vi "Get Main Log Path and Name from Config.vi"(8 "error in":errorcluster, 11 "Main Config File Refnum":T1) -> (0 "error out":errorcluster, 1 "LogBaseName":string, 2 "LogBasePath":path)   [LabVIEW 2018]
uses:
  <vilib>/Utility/config.llb/Config Data RefNum.ctl
  <vilib>/Utility/config.llb/Read Key (String).vi
  <vilib>/Utility/config.llb/NI_LVConfig.lvlib
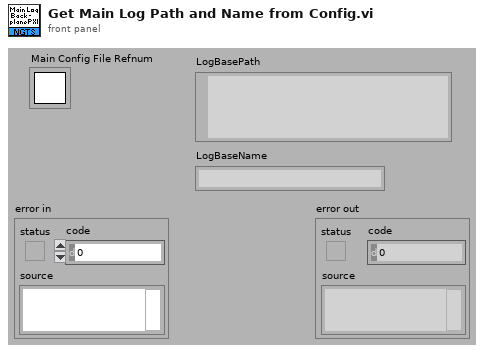
[diagram p1: front panel]
types:
  T1 = typedef "NI_LVConfig.lvlib/Config Data RefNum.ctl" = refnum<k1>
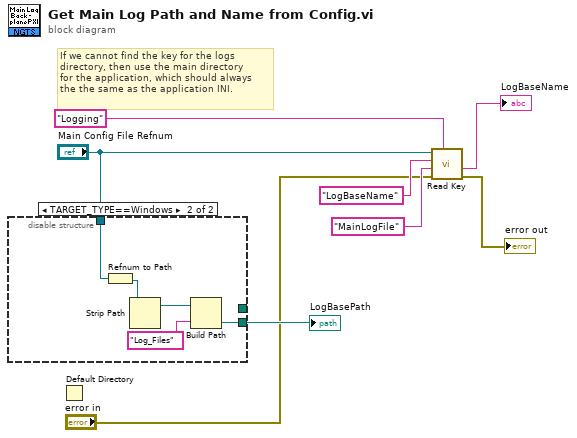
[diagram p0: block diagram]
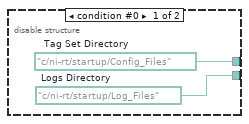
[diagram p2: hidden frame]
diagram:
  # "If we cannot find the key for the logs\ndirectory, then use the main directory\nfor the application, which should always\nthe the same as the application INI."
  n1 = disable-structure shown="TARGET_TYPE==Windows" {
    disable-tunnel: [w10 _] -> _
    disable-tunnel: [w9 w13] -> w3
    disable-tunnel: "Main Config File Refnum" -> [_ w12]
    frame condition #0 {
      w10 = path "c:/ni-rt/startup/Config_Files"  # Tag Set Directory
      w9 = path "c:/ni-rt/startup/Log_Files"  # Logs Directory
    }
    frame condition #1 (active) {
      n2 = Refnum to Path(1:w12) -> (0:w11:path)
      n3 = Strip Path(path=w11) -> (stripped path=w15:path)  [unwired: 1 out]
      n4 = Build Path(base path=w15, name or relative path="Log_Files") -> (appended path=w13:path)
    }
  }
  "LogBasePath" <- w3
  n5 = Default Directory() -> ()  [unwired: 1 out]
  n6 = call-poly <vilib>:"Read Key.vi"("section"="Logging", "error in (no error)"="error in", "default value"="MainLogFile" ("key"), "key"="LogBaseName", "refnum"="Main Config File Refnum") -> ("error out"=→"error out":errorcluster, "value"=→"LogBaseName":string)  [unwired: 3 in, 2 out]
